vi "MIMIC RecvCommand_MP_1.vi"(4 "error in":errorcluster, 7 "VISA resource name":refnum<visa-resource-name>) -> (0 "error out":errorcluster, 1 "Receive_buffer":u8[](array[numeric]), 2 "Receive Buffer_MP":u8[](array[numeric]), 3 "VISA resource name OUT":refnum<visa-resource-name>)   [LabVIEW 2014]
panel:
  out "Index":i32
  out "Num_Bytes":i32
  out "continue_flag":bool=TRUE
  out "STRT_TIME":u32
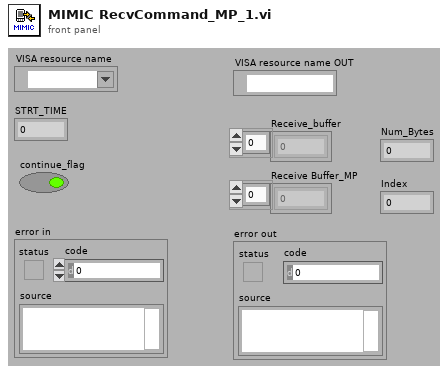
[diagram p1: front panel]
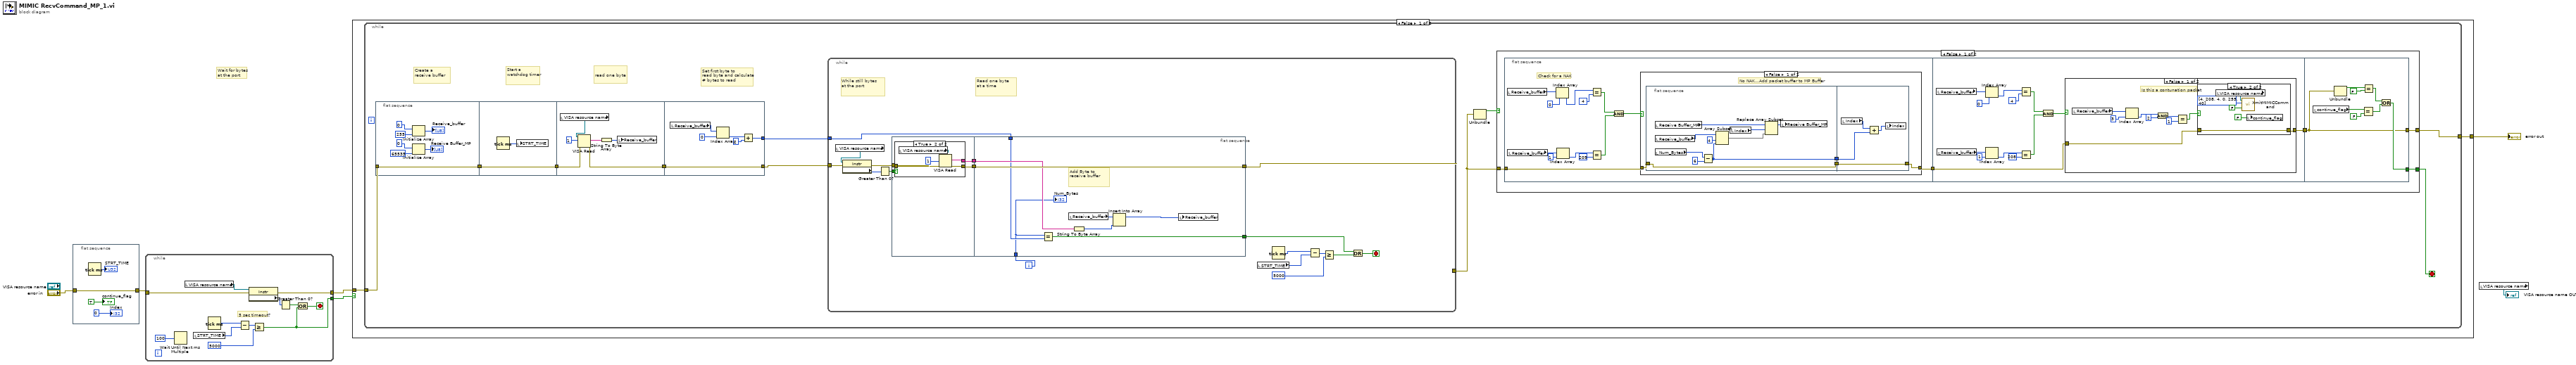
[diagram p0: block diagram]
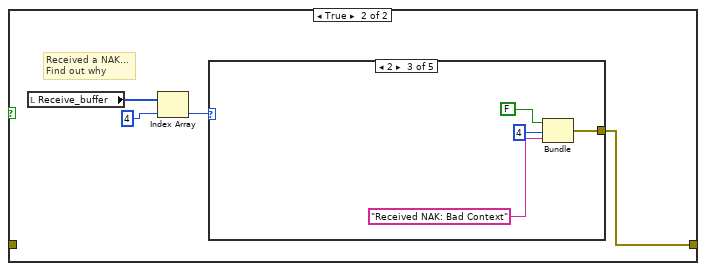
[diagram p2: hidden frame]
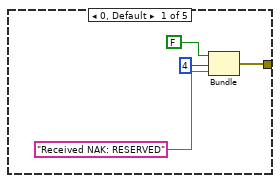
[diagram p3: hidden frame]
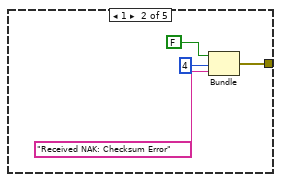
[diagram p4: hidden frame]
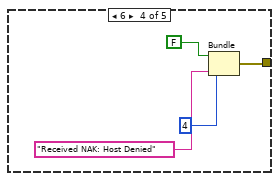
[diagram p5: hidden frame]
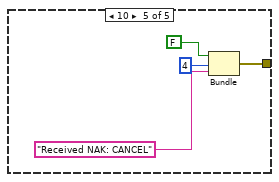
[diagram p6: hidden frame]
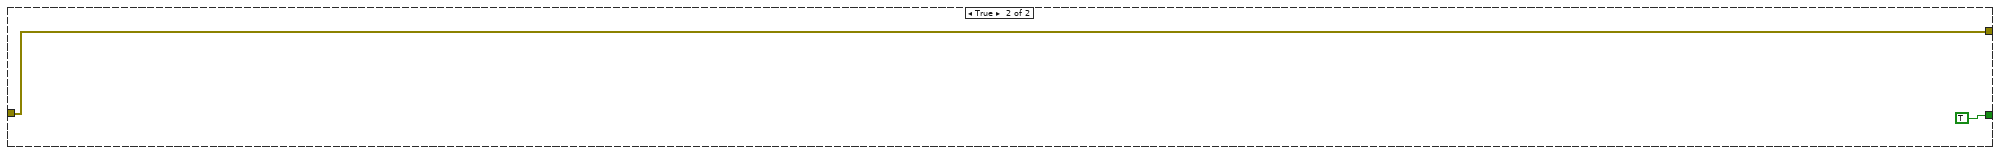
[diagram p9: hidden frame]
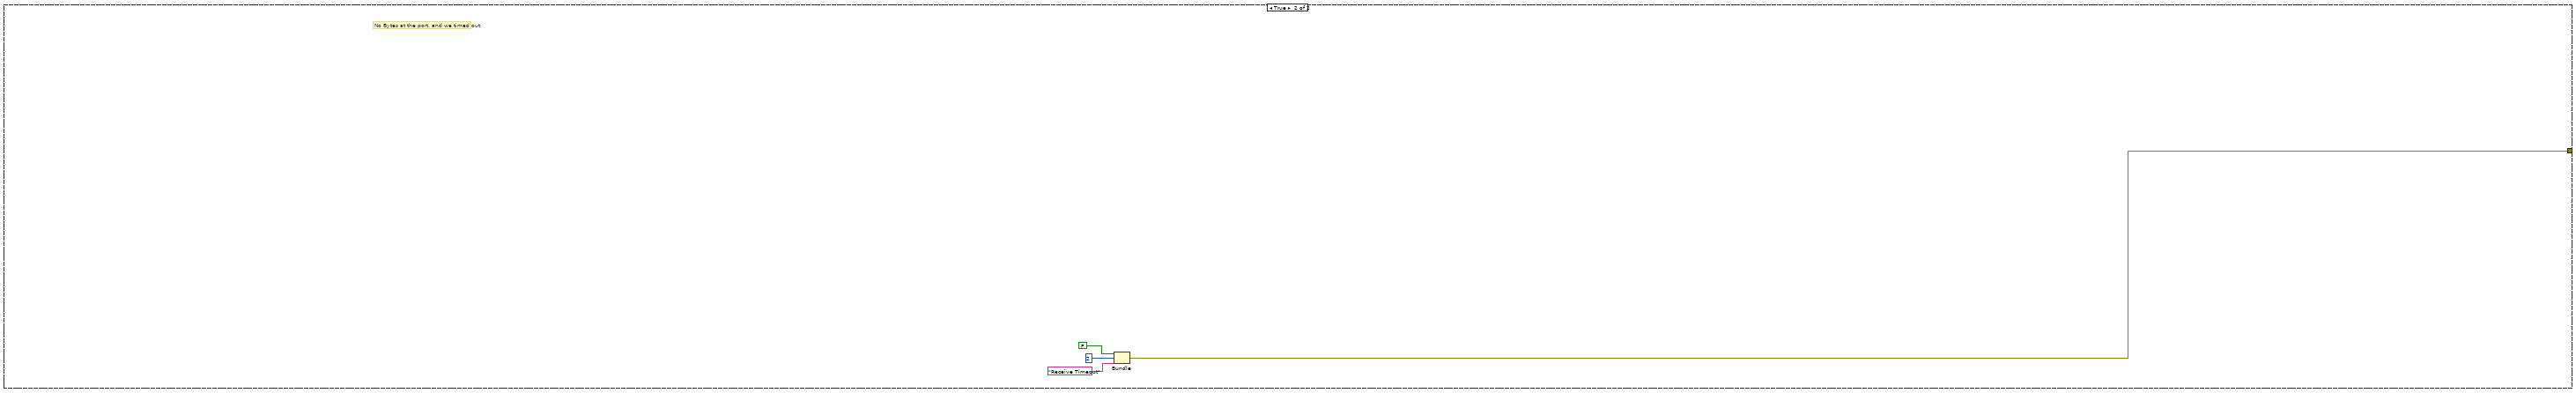
[diagram p11: hidden frame]
diagram:
  # "Wait for bytes\nat the port"
  n1 = flat-sequence {
    tunnel: "error in" -> [w9]
    tunnel: [w9] -> w2
    frame #0 {
      n2 = Tick Count (ms)() -> (millisecond timer value=→"STRT_TIME":u32)
      "continue_flag" <- TRUE
      "Index" <- 0
    }
  }
  n3 = while {
    tunnel: w2 -> [w19]
    tunnel: [w20] -> w6
    tunnel: [w12] -> w5
    stop <- w21 stop-if-true
    # "5 sec timeout?"
    n4 = Wait Until Next ms Multiple(millisecond multiple=u32 100) -> ()  [unwired: 1 out]
    n5 = local read "VISA resource name"() -> (w11:refnum<visa-resource-name>)
    n6 = local read "STRT_TIME"() -> (w13:u32)
    n7 = Tick Count (ms)() -> (millisecond timer value=w16:u32)
    n8 = Subtract(x=w16, y=w13) -> (x-y=w15:u32)
    n9 = property class="Instr"(reference=w11, error in=w19) -> (error out=w20:errorcluster, "Serial Settings:Number of Bytes at Serial Port"=w22:u32)  [unwired: 1 out]
    n10 = Greater Or Equal?(x=w15, y=u32 5000 ("milliseconds to wait")) -> (x >= y?=w12:bool)
    n11 = Greater Than 0?(x=w22) -> (x > 0?=w17:bool)
    n12 = Or(x=w17, y=w12) -> (x .or. y?=w21:bool)
  }
  n13 = case shown="False" w5 {
    tunnel: w6 -> [w24 _]
    tunnel: [w23 w190] -> w4
    frame False {
      n14 = while {
        tunnel: w24 -> [w30]
        tunnel: [w29] -> w23
        stop <- w28 stop-if-true
        # "Start a watchdog timer"
        # "Set first byte to \nread byte and calculate # bytes to read"
        # "read one byte"
        # "Create a\nreceive buffer"
        n15 = flat-sequence {
          tunnel: w30 -> [w140]
          tunnel: [w140] -> w34
          tunnel: w34 -> [w142]
          tunnel: [w142] -> w33
          tunnel: w33 -> [w145]
          tunnel: [w148] -> w27
          tunnel: [w154] -> w31
          tunnel: [w149] -> w32
          tunnel: w27 -> [w154]
          frame #0 {
            n16 = Initialize Array(u8 0 ("element"), 255 ("dimension size")) -> (→"Receive_buffer":u8[])
            n17 = Initialize Array(u8 0 ("element"), 65535 ("dimension size")) -> (→"Receive Buffer_MP":u8[])
          }
          frame #1 {
            n18 = Tick Count (ms)() -> (millisecond timer value=w141:u32)
            n19 = local write "STRT_TIME"(w141) -> ()
          }
          frame #2 {
            n20 = local read "VISA resource name"() -> (w143:refnum<visa-resource-name>)
            n21 = VISA Read(VISA resource name=w143, byte count=u32 1, error in (no error)=w145) -> (read buffer=w147:string, error out=w148:errorcluster)  [unwired: 2 out]
            n22 = String To Byte Array(string=w147) -> (unsigned byte array=w144:u8[])
            n23 = local write "Receive_buffer"(w144) -> ()
          }
          frame #3 {
            n24 = local read "Receive_buffer"() -> (w150:u8[])
            n25 = Index Array(array=w150, index=0) -> (element=w151:u8)
            n26 = Add(x=w151, y=u8 2) -> (x+y=w149:u8)
          }
        }
        n27 = while {
          tunnel: w31 -> [w169]
          tunnel: [w167] -> w25
          tunnel: w32 -> [w158]
          i -> [w157]
          stop <- w162 stop-if-true
          # "Read one byte\nat a time"
          # "While still bytes\nat the port"
          n28 = local read "VISA resource name"() -> (w155:refnum<visa-resource-name>)
          n29 = property class="Instr"(reference=w155, error in=w169) -> (error out=w168:errorcluster, "Serial Settings:Number of Bytes at Serial Port"=w171:u32)  [unwired: 1 out]
          n30 = Greater Than 0?(x=w171) -> (x > 0?=w170:bool)
          n31 = flat-sequence {
            tunnel: w170 -> [w175]
            tunnel: w168 -> [w174]
            tunnel: [w173] -> w160
            tunnel: [w172] -> w159
            tunnel: [w189] -> w167
            tunnel: w160 -> [w185]
            tunnel: w159 -> [w189]
            tunnel: w158 -> [w184]
            tunnel: w157 -> [w182]
            tunnel: [w183] -> w156
            frame #0 {
              n32 = case shown="True" w175 {
                tunnel: w174 -> [w176 w181]
                tunnel: [w176 w180] -> w172
                tunnel: [_ w179] -> w173
                frame False {
                }
                frame True {
                  n33 = local read "VISA resource name"() -> (w177:refnum<visa-resource-name>)
                  n34 = VISA Read(VISA resource name=w177, byte count=u32 1, error in (no error)=w181) -> (read buffer=w179:string, error out=w180:errorcluster)  [unwired: 2 out]
                }
              }
            }
            frame #1 {
              # "Add Byte to \nreceive buffer"
              n35 = Equal?(x=w182, y=w184) -> (x = y?=w183:bool)
              n36 = local read "Receive_buffer"() -> (w187:u8[])
              n37 = String To Byte Array(string=w185) -> (unsigned byte array=w186:u8[])
              n38 = Insert Into Array(array=w187, new element=w186) -> (w188:u8[])  [unwired: 1 in]
              n39 = local write "Receive_buffer"(w188) -> ()
              "Num_Bytes" <- w182
            }
          }
          n40 = local read "STRT_TIME"() -> (w163:u32)
          n41 = Tick Count (ms)() -> (millisecond timer value=w166:u32)
          n42 = Subtract(x=w166, y=w163) -> (x-y=w165:u32)
          n43 = Greater Or Equal?(x=w165, y=u32 5000 ("milliseconds to wait")) -> (x >= y?=w161:bool)
          n44 = Or(x=w156, y=w161) -> (x .or. y?=w162:bool)
        }
        n45 = Unbundle(w25) -> ("status"=w26:bool)  [unwired: 2 out]
        n46 = case shown="False" w26 {
          tunnel: w25 -> [w37 w133]
          tunnel: [w36 w133] -> w29
          tunnel: [w35 TRUE] -> w28
          frame False {
            n47 = flat-sequence {
              tunnel: w37 -> [w41]
              tunnel: [w40] -> w39
              tunnel: w39 -> [w96]
              tunnel: [w95] -> w38
              tunnel: [w124] -> w36
              tunnel: w38 -> [w124]
              tunnel: [w125] -> w35
              frame #0 {
                # "Check for a NAK"
                n48 = local read "Receive_buffer"() -> (w52:u8[])
                n49 = local read "Receive_buffer"() -> (w49:u8[])
                n50 = Index Array(array=w52, index=0) -> (element=w47:u8)
                n51 = Index Array(array=w49, index=1) -> (element=w46:u8)
                n52 = Equal?(x=w47, y=u8 4) -> (x = y?=w48:bool)
                n53 = Equal?(x=w46, y=u8 209) -> (x = y?=w45:bool)
                n54 = And(x=w48, y=w45) -> (x .and. y?=w42:bool)
                n55 = case shown="False" w42 {
                  tunnel: w41 -> [w56 _]
                  tunnel: [w54 w71] -> w40
                  frame False {
                    # "No NAK...Add packet buffer to MP Buffer"
                    n56 = flat-sequence {
                      tunnel: w56 -> [w58]
                      tunnel: [w58] -> w55
                      tunnel: [w57] -> w53
                      tunnel: w55 -> [w69]
                      tunnel: [w69] -> w54
                      tunnel: w53 -> [w67]
                      frame #0 {
                        n57 = local read "Receive Buffer_MP"() -> (w63:u8[])
                        n58 = local read "Receive_buffer"() -> (w65:u8[])
                        n59 = local read "Num_Bytes"() -> (w62:i32)
                        n60 = Subtract(x=w62, y=6) -> (x-y=w57:i32)
                        n61 = Array Subset(array=w65, index=4, length=w57) -> (w60:u8[])
                        n62 = local read "Index"() -> (w59:i32)
                        n63 = Replace Array Subset(array=w63, new element=w60, index=w59) -> (w66:u8[])
                        n64 = local write "Receive Buffer_MP"(w66) -> ()
                      }
                      frame #1 {
                        n65 = local read "Index"() -> (w68:i32)
                        n66 = Add(x=w68, y=w67) -> (x+y=w70:i32)
                        n67 = local write "Index"(w70) -> ()
                      }
                    }
                  }
                  frame True {
                    # "Received a NAK...\nFind out why"
                    n68 = local read "Receive_buffer"() -> (w73:u8[])
                    n69 = Index Array(array=w73, index=4) -> (element=w72:u8)
                    n70 = case shown="2" w72 {
                      tunnel: [w75 w79 w83 w87 w91] -> w71
                      frame 0, Default {
                        n71 = Bundle(FALSE, 4, "Received NAK: RESERVED") -> (w75:errorcluster)  [unwired: 1 in]
                      }
                      frame 1 {
                        n72 = Bundle(FALSE, 4, "Received NAK: Checksum Error") -> (w79:errorcluster)  [unwired: 1 in]
                      }
                      frame 2 {
                        n73 = Bundle(FALSE, 4, "Received NAK: Bad Context") -> (w83:errorcluster)  [unwired: 1 in]
                      }
                      frame 6 {
                        n74 = Bundle(FALSE, 4, "Received NAK: Host Denied") -> (w87:errorcluster)  [unwired: 1 in]
                      }
                      frame 10 {
                        n75 = Bundle(FALSE, 4, "Received NAK: CANCEL") -> (w91:errorcluster)  [unwired: 1 in]
                      }
                    }
                  }
                }
              }
              frame #1 {
                n76 = local read "Receive_buffer"() -> (w101:u8[])
                n77 = local read "Receive_buffer"() -> (w100:u8[])
                n78 = Index Array(array=w101, index=0) -> (element=w99:u8)
                n79 = Index Array(array=w100, index=1) -> (element=w98:u8)
                n80 = Equal?(x=w99, y=u8 4) -> (x = y?=w105:bool)
                n81 = Equal?(x=w98, y=u8 208) -> (x = y?=w104:bool)
                n82 = And(x=w105, y=w104) -> (x .and. y?=w97:bool)
                n83 = case shown="False" w97 {
                  tunnel: w96 -> [w110 w123]
                  tunnel: [w109 w123] -> w95
                  frame False {
                    # "Is this a contunation packet"
                    n84 = local read "Receive_buffer"() -> (w116:u8[])
                    n85 = Index Array(array=w116, index=3) -> (element=w114:u8)
                    n86 = And(x=w114, y=u8 2) -> (x .and. y?=w112:u8)
                    n87 = Equal?(x=w112, y=u8 1) -> (x = y?=w108:bool)
                    n88 = case shown="True" w108 {
                      tunnel: w110 -> [w117 w121]
                      tunnel: [w117 w121] -> w109
                      frame False {
                      }
                      frame True {
                        n89 = local read "VISA resource name"() -> (w118:refnum<visa-resource-name>)
                        n90 = call "XmitMIMICCommand.vi"("HWHSflag"=FALSE, "Command array"=u8[] [4, 208, 4, 0, 255, 40], "VISA resource name"=w118) -> ()  [unwired: 1 in, 2 out]
                        n91 = local write "continue_flag"(FALSE ("continue_flag")) -> ()
                      }
                    }
                  }
                  frame True {
                  }
                }
              }
              frame #2 {
                n92 = local read "continue_flag"() -> (w127:bool)
                n93 = Unbundle(w124) -> ("status"=w129:bool)  [unwired: 2 out]
                n94 = Equal?(x=w127, y=FALSE) -> (x = y?=w126:bool)
                n95 = Equal?(x=w129, y=FALSE) -> (x = y?=w131:bool)
                n96 = Or(x=w131, y=w126) -> (x .or. y?=w125:bool)
              }
            }
          }
          frame True {
          }
        }
      }
    }
    frame True {
      # "No Bytes at the port, and we timed out"
      n97 = Bundle(FALSE, 2, "Receive Timeout") -> (w190:errorcluster)  [unwired: 1 in]
    }
  }
  "error out" <- w4
  n98 = local read "VISA resource name"() -> (→"VISA resource name OUT":refnum<visa-resource-name>)
